vi "16进制字符串至可视化ASIIC字符串.vi"(7 "字节分隔符(无)":string, 11 "十六进制字符串":string) -> (3 "可视化16进制":string)   [LabVIEW 2013]
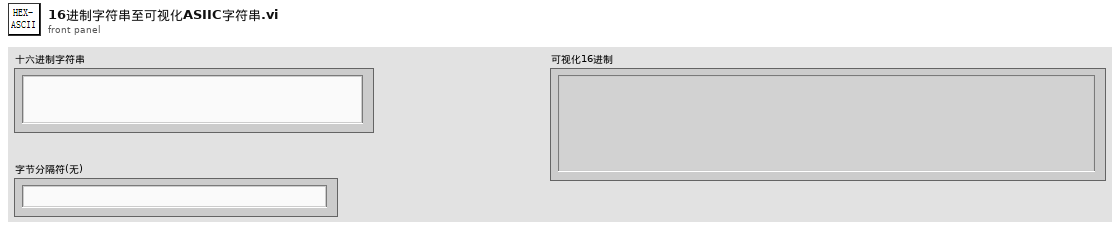
[diagram p1: front panel]
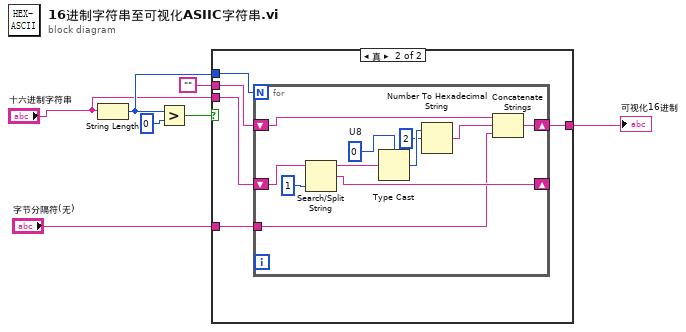
[diagram p0: block diagram]
diagram:
  n1 = String Length(string="十六进制字符串") -> (length=w5:i32)
  n2 = Greater?(x=w5, y=0) -> (0:w3:bool)
  n3 = case shown="真" w3 {
    tunnel: w5 -> [_ w12]
    tunnel: "十六进制字符串" -> [_ w11]
    tunnel: [_ w10] -> w7
    tunnel: "" -> [_ w9]
    tunnel: "字节分隔符(无)" -> [_ w8]
    frame False {
    }
    frame True {
      n4 = for {
        N: w12 -> [_]
        shift-right: [w17] -> _
        shift-left: w11 -> [w18]
        shift-right: [w16] -> w10
        shift-left: w9 -> [w15]
        tunnel: w8 -> [w13]
        w21 = u8 0  # U8
        n5 = Search/Split String(string=w18, offset (0)=1 ("偏移量(0)")) -> (substring before match=w23:string, match + rest of string=w17:string)  [unwired: 1 in, 1 out]
        n6 = Type Cast(type=w21, x=w23) -> (*(type *) &x=w20:u8)
        n7 = Number To Hexadecimal String(1:i16 2 ("宽度(-)"), 2:w20) -> (0:w19:string)
        n8 = Concatenate Strings(w15, w19, w13) -> (w16:string)
      }
    }
  }
  "可视化16进制" <- w7
